vi "DO Data's.vi"(8 "error in":errorcluster, 10 "DO Data's":T1, 11 "Module ID":i32=-1) -> (0 "error out":errorcluster)   [LabVIEW 2021, in "RT Acquisition Engine.lvlib"]
doc: "This Broadcast event will send DO data's to all the module's which regester's this event refnum.\n_____\nCreated using DQMH Event Scripter 7.0.1.1316."
uses:
  RT Acquisition Engine.lvlib
  Host-Control's/DIO Data's from RT.ctl
  DO Data's Argument--cluster.ctl
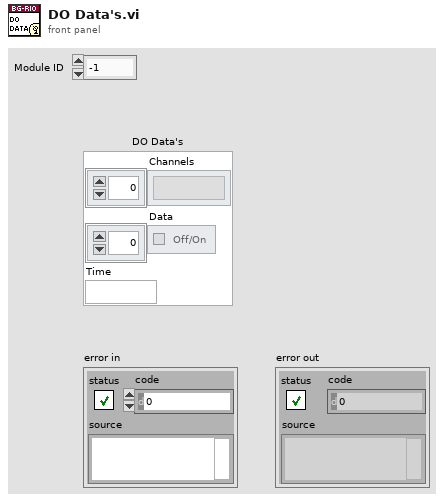
[diagram p1: front panel]
types:
  T1 = typedef "DIO Data's from RT.ctl" = cluster{"Channels":string[], "Data":bool[], "Time":string}
  T2 = typedef "RT Acquisition Engine.lvlib/DO Data's Argument--cluster.ctl" = cluster{"Module ID":i32, "DO Data's":T1}
  T3 = typedef "RT Acquisition Engine.lvlib/Broadcast Events--cluster.ctl" = cluster{"Module Did Init":refnum<user-event>, "Status Updated":refnum<user-event>, "Error Reported":refnum<user-event>, "Module Did Stop":refnum<user-event>, "Update Module Execution Status":refnum<user-event>, "RT Connection Status":refnum<user-event>, "Tx RT Hardware Info":refnum<user-event>, "DO Data's":refnum<user-event>}
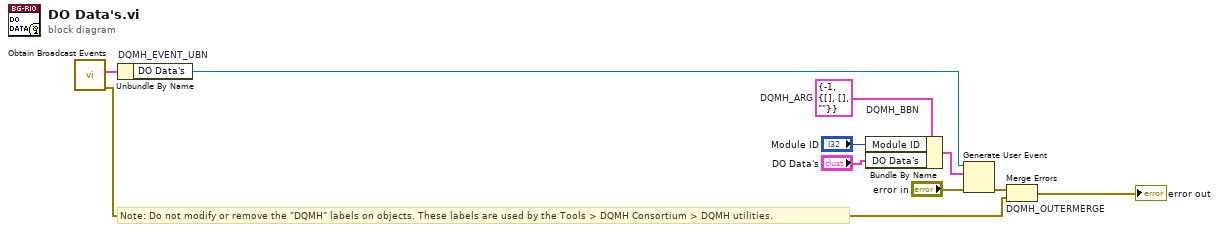
[diagram p0: block diagram]
diagram:
  w5 = T2 {"Module ID"=-1, "DO Data's"={"Channels"=[], "Data"=[], "Time"=""}}  # DQMH_ARG
  # "Note: Do not modify or remove the \"DQMH\" labels on objects. These labels are used by the Tools > DQMH Consortium > DQMH utilities."
  n1 = call "Obtain Broadcast Events.vi"() -> ("error out"=w2:errorcluster, "RT Acquisition Engine Broadcast Events"=w1:T3)  [unwired: 10 in]
  n2 = Unbundle By Name "DQMH_EVENT_UBN"(w1) -> ("DO Data's"=w7:refnum<user-event>)
  n3 = Bundle By Name "DQMH_BBN"(cluster=w5, "Module ID"="Module ID", "DO Data's"="DO Data's") -> (w8:T2)
  n4 = Generate User Event(user event=w7, event data cluster=w8, error in="error in") -> (error out=w6:errorcluster)  [unwired: 1 in, 1 out]
  n5 = Merge Errors "DQMH_OUTERMERGE"(w6, w2) -> (→"error out":errorcluster)
